vi "Scope_5782.vi"() -> ()   [LabVIEW 2013]
uses:
  <vilib>/userdefined/High Color/nirio_resource_hc.ctl
  FPGA/DataMode.ctl
  <vilib>/Analysis/4window.llb/windowTd.ctl
  Host/Scope/controls/power_spectrum_unit.ctl
  Host/Scope5782/Scope/controls/5782_trigger_type.ctl
  Host/Scope/controls/Data_calc_mode.ctl
  Host/Scope/controls/Data_display_mode.ctl
  Host/Scope/controls/Graph_references.ctl
  Host/Scope/controls/graph_controls.ctl
  Host/Scope/controls/Channel_select.ctl
  Host/Scope5782/Config/FPGAref_5782.ctl
  Host/Communication/response.ctl
  Host/Communication/driver_status.ctl
  Host/Communication/Driver/RemoteConnection/RemoteReferences.ctl
  Host/Communication/Driver/TcpServerDriver/TcpServerDriver.lvclass
  Host/Scope/controls/ScopeMode.ctl
  FPGA/fpga_settings.ctl
  Host/Communication/global_stop.vi
  <vilib>/FPGAPlugInAG/PXIe-7975R/niLvFpga_Open_PXIe-7975R.vi
  <vilib>/rvi/interface/common/dynamic/niFpgaDynamicAddResources.vi
  <vilib>/rvi/interface/common/niFpgaWaitOnOcc.vi
  <vilib>/Utility/error.llb/Error Cluster From Error Code.vi
  <vilib>/rvi/errors/niLvFpgaAdjustHostInterfaceError.vi
  <vilib>/FPGAPlugInAG/Dynamic/niLvFpga_Close_Dynamic.vi
  <vilib>/rvi/interface/nirviOpenFPGA/nirviOpenFPGA.xnode
  FPGA Bitfiles/mixer_FPGATarget2_FPGAmain5782_W462Q9ePIkg.lvbitx
  <vilib>/rvi/interface/nirviReadWriteControl/nirviReadWriteControl.xnode
  <vilib>/rvi/FXPMathLib/FxpInterpret/XNode/nifxpmath_Interpret.xnode
  <vilib>/rvi/interface/nirviCloseFPGA/nirviCloseFPGA.xnode
  Host/Utilities/Ticker/Ticker.lvclass
  NiFpgaLv.dll
  <vilib>/rvi/interface/Simulation/niFpgaSimulationCallBeginRW.vi
  Host/Communication/Driver/RemoteConnection/RemoteConnection.lvclass
  <vilib>/Analysis/NI_AALPro.lvlib
panel:
  in  "deltaF":bool
  in  "b":fxp<+/-,16,2>
  in  "a":fxp<+/-,16,2>
  in  "Fequency [kHz]":dbl format="%#_8g"
  in  "#bins":i32=1 min=1 max=16
  in  "ch1 DC offset":dbl caption="DC offset\nChannel 1"
  in  "ch0 DC offset":dbl caption="DC offset\nChannel 0"
  in  "Output delay delta":dbl(slide) scale=0.0..6.0
  in  "Output delay":dbl(slide) scale=0.0..6.0
  in  "Chart length":i32=200000
  in  "Trigmode":enum32{"Triggered", "Continuous"}(radio)
  in  "Refence for phase":T1
  in  "Graph_refs":T2
  out "Lower chart":dbl[][](graph)
  out "Upper chart":dbl[][](graph)
  out "Lower graph":i16[][](graph)
  in  "Buffer":T4
  in  "Display":T5
  in  "Output mixer fequency [MHz]":dbl
  in  "Trigger":T6
  in  "Ch1 Q":bool
  in  "Ch1 I":bool
  in  "Ch0 Q":bool
  in  "Ch0 I":bool
  in  "Ch1":bool
  in  "Ch0":bool
  out "stop 2":bool
  in  "Zoom freq X":bool
  in  "Zoom freq Y":bool
  in  "Zoom time Y":bool
  in  "Zoom time X":bool
  in  "Unit":T7
  in  "Window":T8=1 items=["Rectangle"=0, "Hanning"=1, "Hamming"=2, "Blackman-Harris"=3, "Exact Blackman"=4, "Blackman"=5, "Flat Top"=6, "4 Term B-Harris "=7, "7 Term B-Harris"=8, "Low Sidelobe"=9, "Blackman Nuttall"=11, "Triangle"=30, "Bartlett-Hanning"=31, "Bohman"=32, "Parzen"=33, "Welch"=34, "Kaiser"=60, "Dolph-Chebyshev"=61, "Gaussian"=62]
  in  "Samples per 5782 record":i32
  in  "Phase offset (deg)":dbl
  in  "Fequency [MHz]":dbl format="%#_8g"
  in  "Mode":T9
  in  "Mixer freq [MHz]":dbl
  out "freqdata":cluster{"f0":dbl, "df":dbl, "magnitude":dbl[]}[](graph)
  in  "Rumode":bool
  in  "Singleshot":bool
  out "error IO":errorcluster
  in  "stop":bool
  in  "resource name":T10="RIO0"
  out "Clocking Option Configured?":bool
  out "Configured?":bool
  # "FPGA setup"
  # "V"
  # "V"
  # "Output delay"
  # "ns"
  # "Auto Zoom"
  # "Output delay delta"
  # "ps"
  # "5782"
  # "Amplitude modulation"
  # "Simulated data"
  # "FFT"
  # "Auto Zoom"
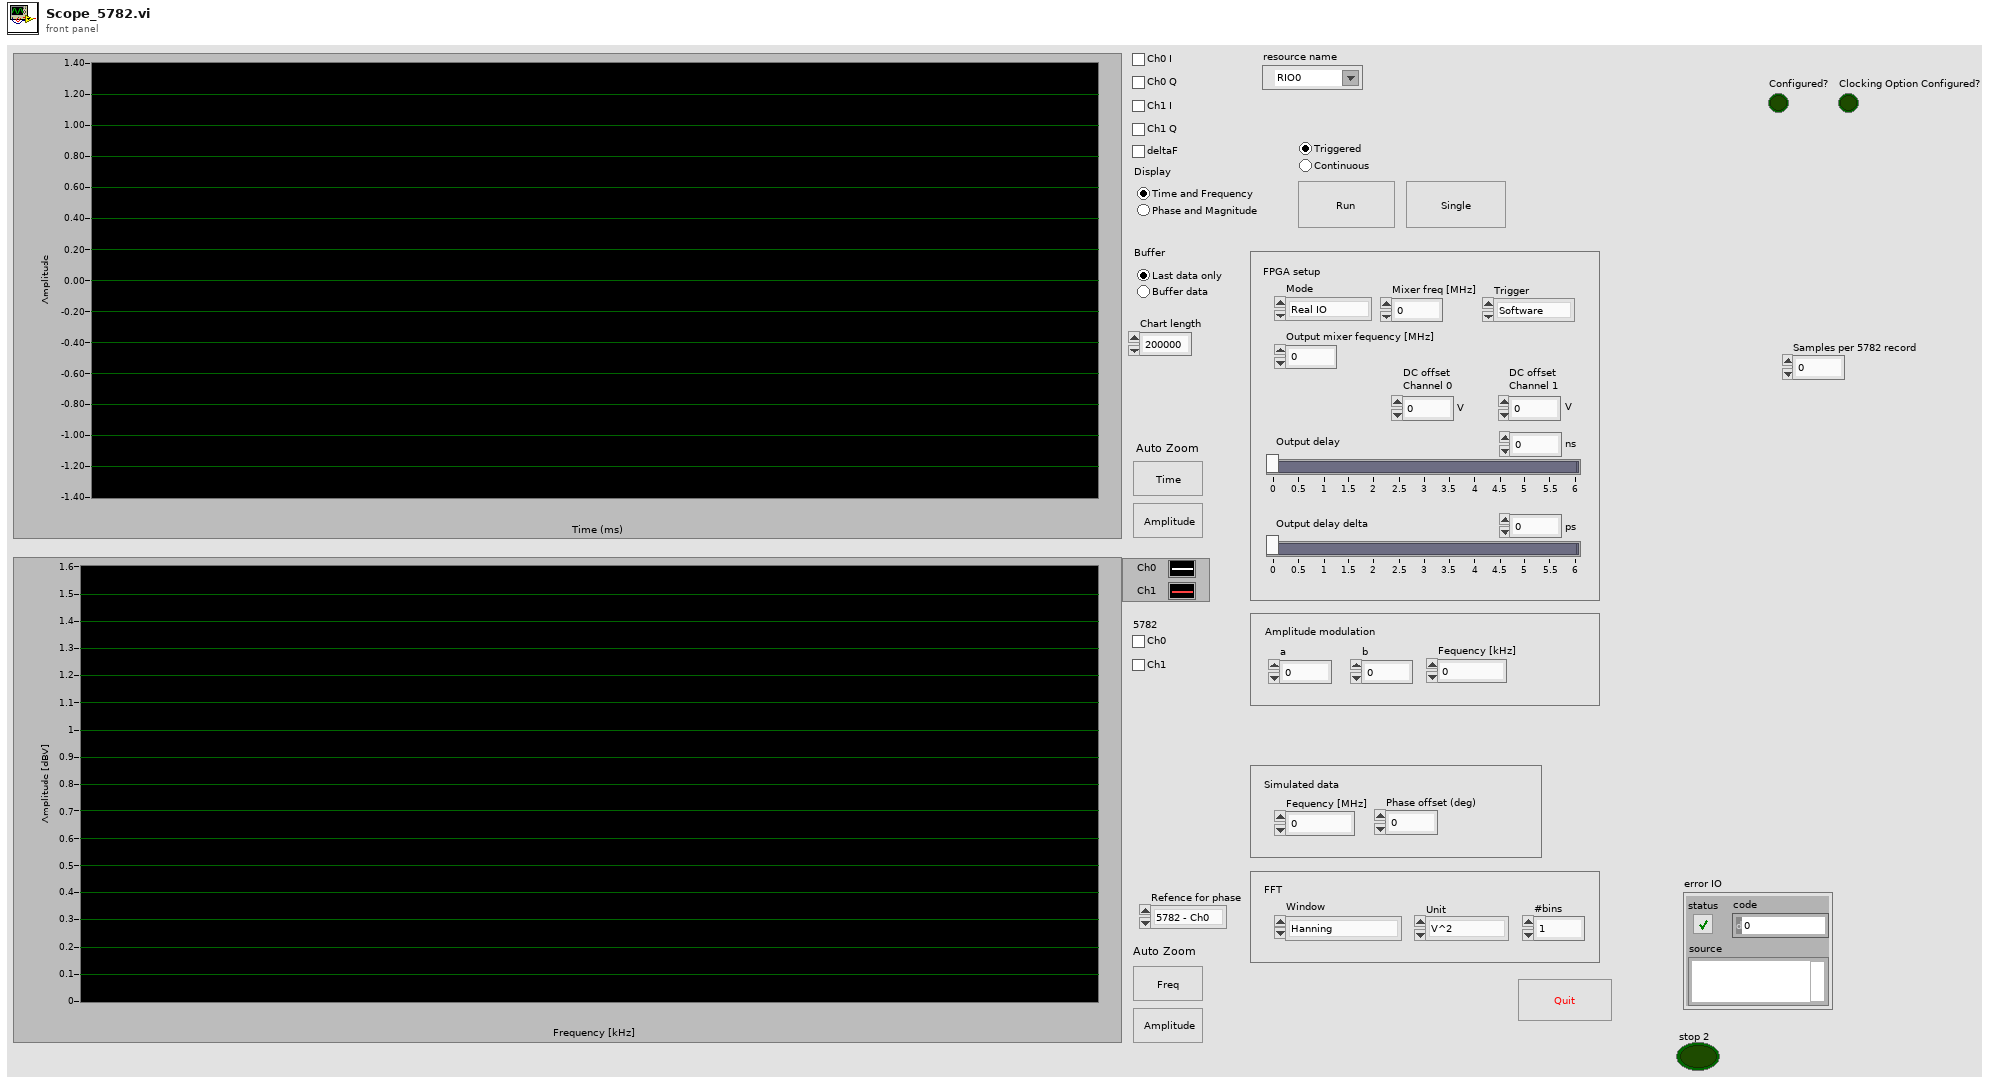
[diagram p1: front panel]
types:
  T1 = typedef "Channel_select.ctl" = enum16{"5782 - Ch0", "5782 - Ch1"}
  T2 = typedef "Graph_references.ctl" = cluster{"upper":T3, "lower":T3, "Freq graph":refnum<vi>}
  T3 = typedef "graph_controls.ctl" = cluster{"Graph":refnum<vi>, "Time btn":refnum<vi>, "Amplitude btn":refnum<vi>, "Chart":refnum<vi>}
  T4 = typedef "Data_display_mode.ctl" = enum32{"Last data only", "Buffer data"}
  T5 = typedef "Data_calc_mode.ctl" = enum32{"Time and Frequency", "Phase and Magnitude"}
  T6 = typedef "5782_trigger_type.ctl" = enum16{"Software", "Trigger input"}
  T7 = typedef "power_spectrum_unit.ctl" = enum16{"V^2", "V", "dBV"}
  T8 = typedef "NI_AALPro.lvlib/windowTd.ctl" = u32
  T9 = typedef "DataMode.ctl" = enum16{"Real IO", "Simulated"}
  T10 = typedef "nirio_resource_hc.ctl" = tag
  T11 = typedef "RemoteConnection.lvclass/RemoteReferences.ctl" = cluster{"a":refnum<vi>, "b":refnum<vi>, "fm":refnum<vi>}
  T12 = typedef "response.ctl" = cluster{"driver status":T13, "Sender":string, "Type":i32, "Variant":variant}
  T13 = typedef "driver_status.ctl" = enum16{"Normal", "Startup", "Connection lost", "Reconnected", "Timeout", "Idle", "Busy"}
  T14 = typedef "FPGAref_5782.ctl" = refnum<k20>
  T15 = enum8{"Internal Clock PLL Off", "Internal Clock PLL On (REF IN)", "External Clock (CLK_IN)", "Internal Clock PLL On (IoModSyncClk)"}
  T16 = typedef "message_queue.ctl" = refnum<queue>
  T17 = typedef "scope_params_5782.ctl" = cluster{"scope mode":T18, "ticker":refnum<class "Ticker.lvclass">, "samples per record":i32, "FPGA ref":T14, "data mode":T9, "5782 Trigger":T6, "Chart length":i32, "RemoteConnection":refnum<class "RemoteConnection.lvclass">, "last phase":dbl[]}
  T18 = typedef "ScopeMode.ctl" = enum16{"Stopped", "Single", "Running", "Continuous"}
  T19 = typedef "fpga_settings.ctl" = enum16{"Feedback Enable", "New FIR coeffs", "FIR shift", "Enable filter", "Set Downsample", "Downsample", "CIC Gain", "Record length", "Trigger samples", "Quiet time", "a_am", "b_am", "Use fixed delay", "fixed sin_fi", "fixed cos_fi", "Ki*Tau", "Kp", "Kd_Tau", "Fi_start", "Fi_delta", "DC_offs 0", "DC_offs 1"}
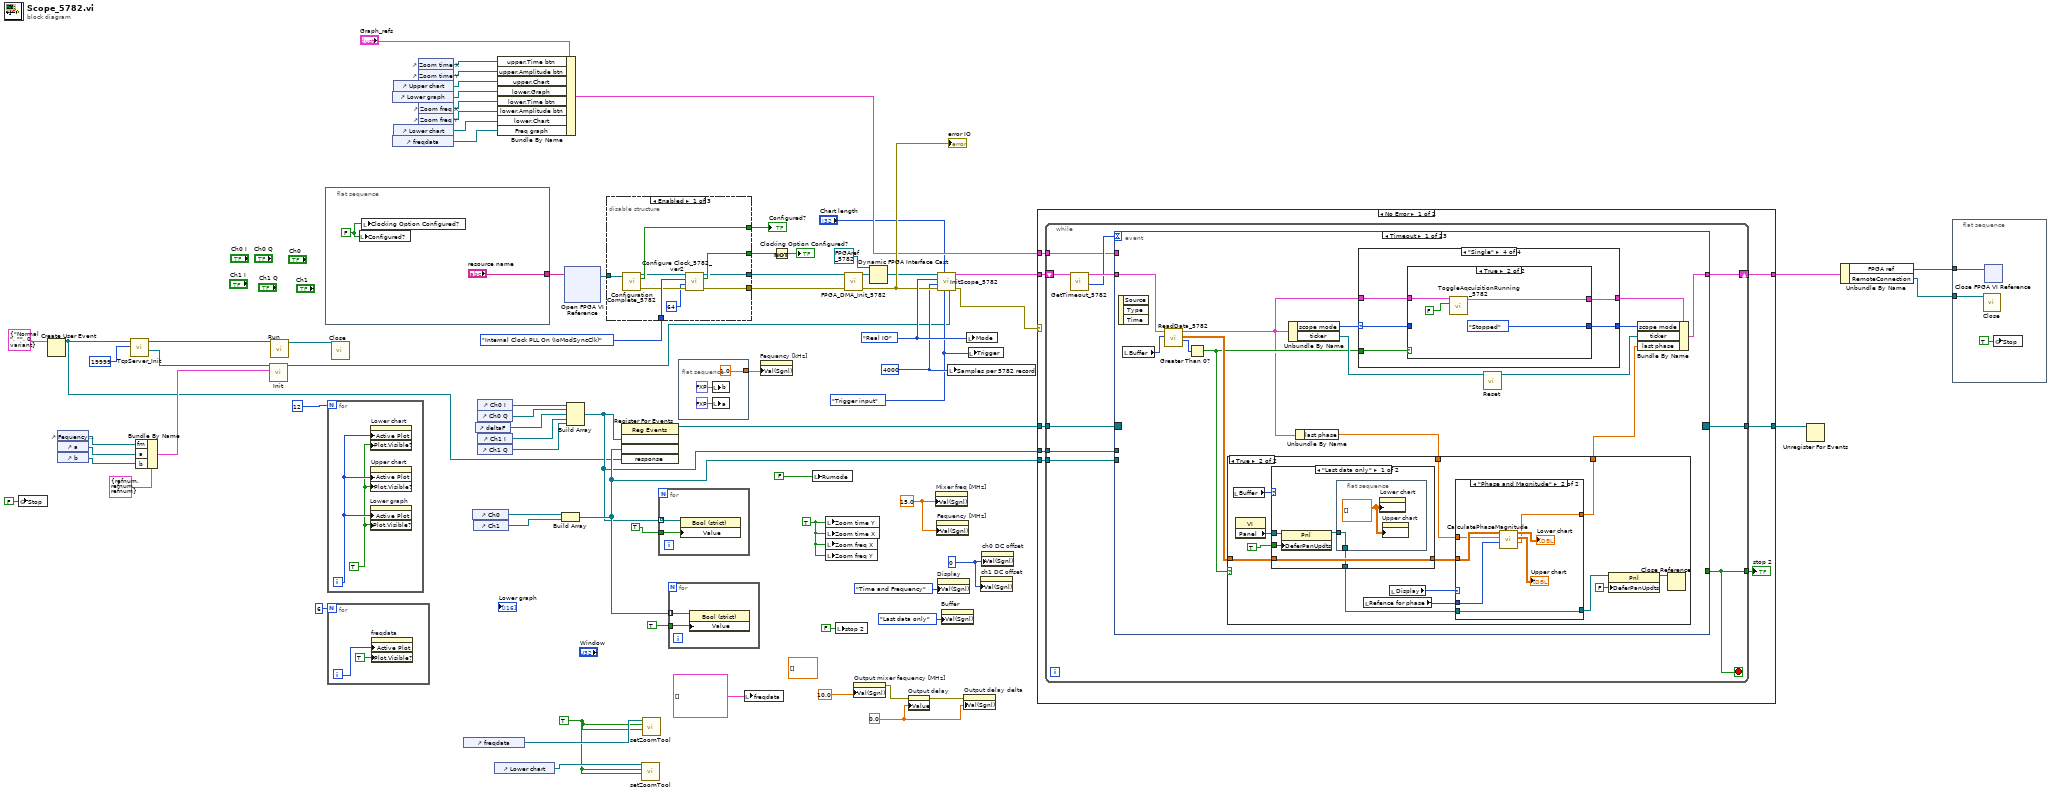
[diagram p0: block diagram]
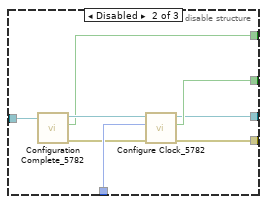
[diagram p2: hidden frame]
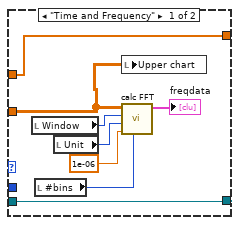
[diagram p6: hidden frame]
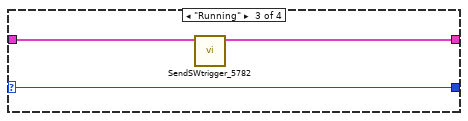
[diagram p9: hidden frame]
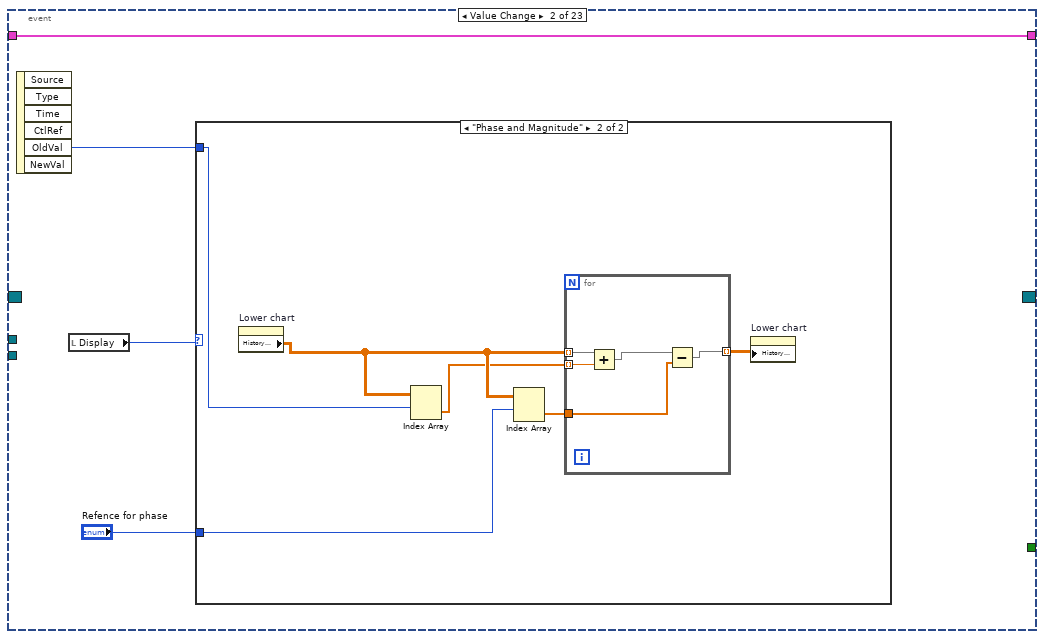
[diagram p11: hidden frame]
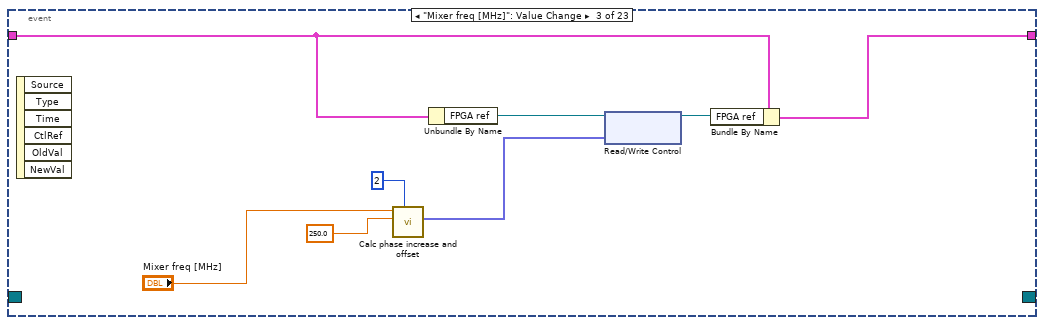
[diagram p13: hidden frame]
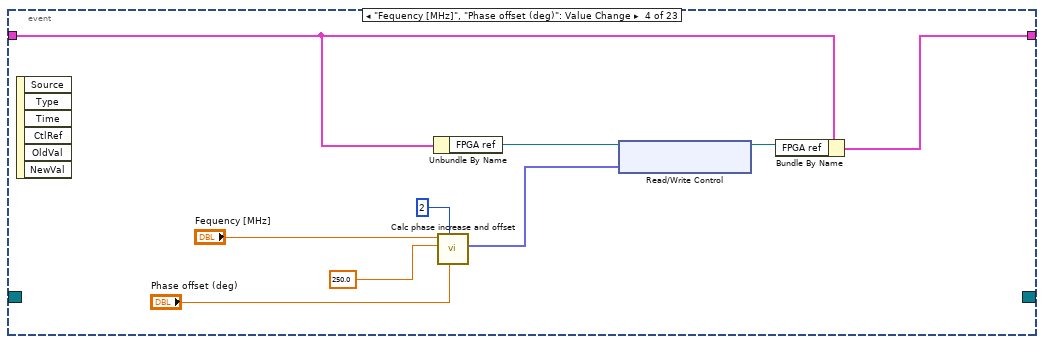
[diagram p14: hidden frame]
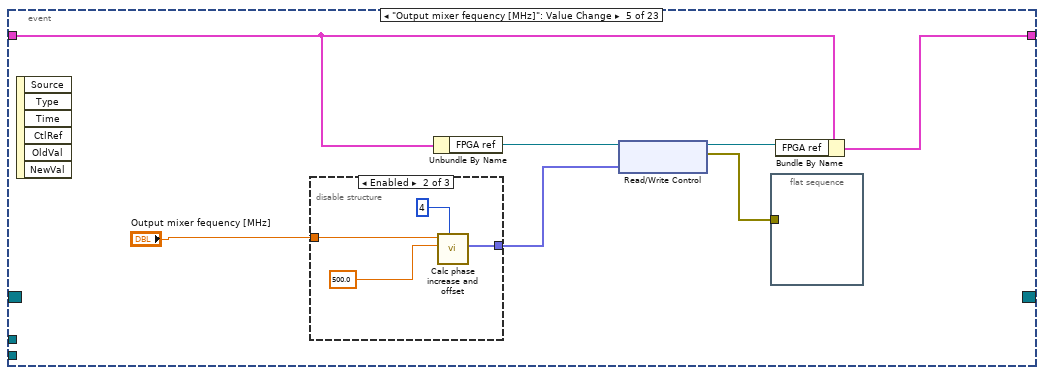
[diagram p15: hidden frame]
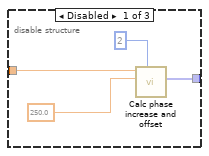
[diagram p16: hidden frame]
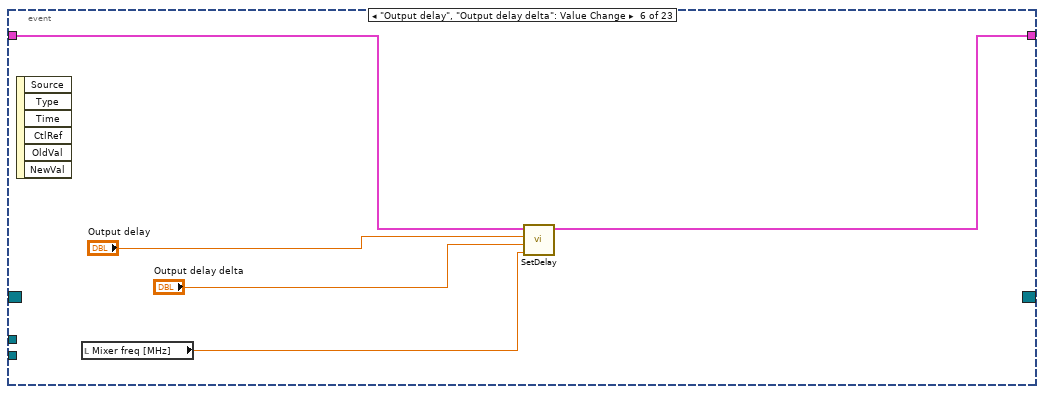
[diagram p18: hidden frame]
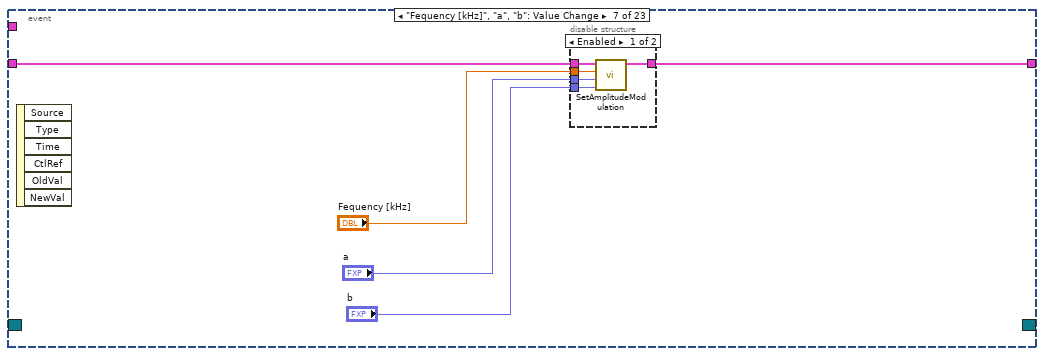
[diagram p19: hidden frame]
diagram:
  w26 = i16 0 ("Value (Signaling)")
  w27 = 0.0 ("Value (Signaling)")
  w49 = 5782_trigger_type."Trigger input" ("Trigger")
  w2 = TRUE ("Zoom  X")
  w62 = TRUE ("Rumode")
  w61 = DataMode."Real IO" ("Mode")
  w50 = 4000 ("Samples to aqcuire")
  (unwired) dbl[][] [] ("Timedata")
  w72 = 15.0 ("Mixer requency [MHz]")
  n1 = global write "global_stop.vi" "Stop"(FALSE ("Stop")) -> ()
  n2 = Create User Event(user event datatype=T12 {"driver status"=enum."Normal", "Sender"="", "Type"=0, "Variant"=variant} ("response")) -> (user event=w9:refnum<user-event>)  [unwired: 1 in, 1 out]
  n3 = control-ref of="Fequency [kHz]"() -> (w12:refnum<vi>)
  n4 = control-ref of="a"() -> (w11:refnum<vi>)
  n5 = control-ref of="b"() -> (w10:refnum<vi>)
  n6 = call "TcpServer_Init.vi"("local port"=u16 19999, "response event"=w9) -> ("Message queue"=w19:T16, "TcpServerDriver"=w16:refnum<class "TcpServerDriver.lvclass">)  [unwired: 8 in]
  n7 = Bundle By Name(cluster=T11 {"a"=refnum, "b"=refnum, "fm"=refnum} ("refs"), "fm"=w12, "a"=w11, "b"=w10) -> (w13:T11)
  n8 = call "Init.vi"("refs"=w13, "server queue"=w19) -> ("RemoteConnection"=w8:refnum<class "RemoteConnection.lvclass">)  [unwired: 9 in]
  n9 = call-dynamic "Run.vi"("BaseDriver in"=w16) -> ("BaseDriver out"=w17:refnum<class "TcpServerDriver.lvclass">)  [unwired: 9 in, 1 out]
  n10 = flat-sequence {
    tunnel: ["resource name"] -> w63
    frame #0 {
      w76 = FALSE ("Trigger Acquisition")
      n11 = local write "Configured?"(w76) -> ()
      n12 = local write "Clocking Option Configured?"(w76) -> ()
    }
  }
  n13 = for {
    N: 12 -> [_]
    i -> [w79]
    w78 = TRUE ("Plot.Visible")
    n14 = property on="Lower graph" class="WFGraph (strict)"("Active Plot"=w79, "Plot.Visible?"=w78) -> ()  [unwired: 2 in, 2 out]
    n15 = property on="Lower chart" class="WFChart (strict)"("Active Plot"=w79, "Plot.Visible?"=w78) -> ()  [unwired: 2 in, 2 out]
    n16 = property on="Upper chart" class="WFChart (strict)"("Active Plot"=w79, "Plot.Visible?"=w78) -> ()  [unwired: 2 in, 2 out]
  }
  n17 = for {
    N: 6 -> [_]
    i -> [w80]
    n18 = property on="freqdata" class="WFGraph (strict)"("Active Plot"=w80, "Plot.Visible?"=TRUE ("Plot.Visible")) -> ()  [unwired: 2 in, 2 out]
  }
  n19 = call-dynamic "Close.vi"("BaseDriver in"=w17) -> ()  [unwired: 9 in, 2 out]
  n20 = control-ref of="Lower graph"() -> (w43:refnum<vi>)
  n21 = control-ref of="freqdata"() -> (w39:refnum<vi>)
  n22 = control-ref of="Upper chart"() -> (w44:refnum<vi>)
  n23 = control-ref of="Lower chart"() -> (w40:refnum<vi>)
  n24 = control-ref of="Zoom time X"() -> (w46:refnum<vi>)
  n25 = control-ref of="Zoom time Y"() -> (w45:refnum<vi>)
  n26 = control-ref of="Zoom freq X"() -> (w42:refnum<vi>)
  n27 = control-ref of="Zoom freq Y"() -> (w41:refnum<vi>)
  n28 = control-ref of="freqdata"() -> (w52:refnum<vi>)
  n29 = control-ref of="Ch0"() -> (w58:refnum<vi>)
  n30 = control-ref of="Ch1"() -> (w59:refnum<vi>)
  n31 = control-ref of="deltaF"() -> (w1:refnum<vi>)
  n32 = control-ref of="Ch0 I"() -> (w54:refnum<vi>)
  n33 = control-ref of="Ch0 Q"() -> (w55:refnum<vi>)
  n34 = control-ref of="Ch1 I"() -> (w56:refnum<vi>)
  n35 = control-ref of="Ch1 Q"() -> (w57:refnum<vi>)
  n36 = control-ref of="Lower chart"() -> (w3:refnum<vi>)
  n37 = Bundle By Name(cluster="Graph_refs", "upper.Time btn"=w46, "upper.Amplitude btn"=w45, "upper.Chart"=w44, "lower.Graph"=w43, "lower.Time btn"=w42, "lower.Amplitude btn"=w41, "lower.Chart"=w40, "Freq graph"=w39) -> (w38:T2)
  n38 = Build Array(w58, w59) -> (w65:refnum<vi>[])
  n39 = xnode "Open FPGA VI Reference"("resource name"=w63) -> ("FPGA VI Reference Out"=w32:refnum<k20>)  [unwired: 1 in, 1 out]
  n40 = Build Array(w54, w55, w1, w56, w57) -> (w53:refnum<vi>[])
  n41 = disable-structure shown="Enabled" {
    disable-tunnel: [w90 w98 _] -> w34
    disable-tunnel: T15."Internal Clock PLL On (IoModSyncClk)" ("Clock Source") -> [w89 w97 _]
    disable-tunnel: [w87 w95 _] -> w33
    disable-tunnel: [w86 w92 w99] -> w25
    disable-tunnel: w32 -> [w83 w94 w99]
    disable-tunnel: [w85 w91 _] -> w30
    frame Enabled {
      n42 = call "Configuration Complete_5782.vi"("FPGA VI Reference in"=w83) -> ("error out"=w88:errorcluster, "Configured?"=w85:bool, "FPGA VI Reference out"=w84:refnum<k20>)  [unwired: 8 in]
      n43 = call "Configure Clock_5782_ver2.vi"("error in"=w88, "User Data 1"=u8 64, "Clock Source"=w89, "FPGA VI Reference"=w84) -> ("error out"=w87:errorcluster, "Configuration Error"=w90:bool, "FPGA VI Reference out"=w86:refnum<k20>)  [unwired: 5 in]
    }
    frame Disabled {
      n44 = call "Configuration Complete_5782.vi"("FPGA VI Reference in"=w94) -> ("error out"=w96:errorcluster, "Configured?"=w91:bool, "FPGA VI Reference out"=w93:refnum<k20>)  [unwired: 8 in]
      n45 = call "Configure Clock_5782.vi"("error in"=w96, "Clock Source"=w97, "FPGA VI Reference in"=w93) -> ("error out"=w95:errorcluster, "Configuration Error"=w98:bool, "FPGA VI Reference Out"=w92:T14)  [unwired: 6 in]
    }
    frame Disabled {
    }
  }
  "Configured?" <- w30
  n46 = register-events(w53, w65, w9) -> (reference out=w69:refnum<event-registration>)  [unwired: 2 in, 1 out]
  n47 = call "setZoomTool.vi"("Zoom Y"=w2, "Zoom  X"=w2, "reference"=w3) -> ()  [unwired: 9 in]
  n48 = call "setZoomTool.vi"("Zoom Y"=w2, "Zoom  X"=w2, "reference"=w52) -> ()  [unwired: 9 in]
  n49 = for {
    tunnel: w53 -> [w101] mode=indexing
    tunnel: TRUE ("Rumode") -> [w100]
    n50 = property class="Bool (strict)"(reference=w101, "Value"=w100) -> ()  [unwired: 1 in, 2 out]
  }
  n51 = for {
    tunnel: w65 -> [w103] mode=indexing
    tunnel: TRUE ("Rumode") -> [w102]
    n52 = property class="Bool (strict)"(reference=w103, "Value"=w102) -> ()  [unwired: 1 in, 2 out]
  }
  n53 = flat-sequence {
    tunnel: [1.0 ("Value (Signaling)")] -> w24
    frame #0 {
      n54 = local write "b"(fxp<+/-,16,2> 0.0 ("b")) -> ()
      n55 = local write "a"(fxp<+/-,16,2> 1.0 ("a")) -> ()
    }
  }
  n56 = local write "freqdata"(cluster{"f0":dbl, "df":dbl, "magnitude":dbl[]}[] [] ("freqdata")) -> ()
  n57 = property on="Fequency [kHz]" class="DigNum (strict)"("Val(Sgnl)"=w24) -> ()  [unwired: 2 in, 2 out]
  n58 = Not(x=w34) -> (.not. x?=→"Clocking Option Configured?":bool)
  n59 = local write "Rumode"(FALSE ("Rumode")) -> ()
  n60 = local write "Zoom time Y"(w62) -> ()
  n61 = local write "Zoom time X"(w62) -> ()
  n62 = local write "Zoom freq X"(w62) -> ()
  n63 = local write "Zoom freq Y"(w62) -> ()
  n64 = local write "stop 2"(FALSE ("stop 2")) -> ()
  n65 = call "FPGA_DMA_Init_5782.vi"("error in (no error)"=w33, "FPGA VI Reference"=w25) -> ("error out"=w51:errorcluster, "FPGA VI Out"=w22:refnum<k20>)  [unwired: 7 in, 1 out]
  "error IO" <- w51
  n66 = property on="Output mixer fequency [MHz]" class="DigNum (strict)"("Val(Sgnl)"=10.0 ("Mixer requency [MHz]")) -> (error out=w28:errorcluster)  [unwired: 2 in, 1 out]
  n67 = Dynamic FPGA Interface Cast(Session In=T14 refnum ("FPGA ref"), Type=w22) -> (Session Out=w21:T14)
  n68 = property on="Output delay" class="Slide (strict)"(error in=w28, "Value"=w27) -> (error out=w29:errorcluster)  [unwired: 1 in, 1 out]
  n69 = property on="Mixer freq [MHz]" class="DigNum (strict)"("Val(Sgnl)"=w72) -> ()  [unwired: 2 in, 2 out]
  n70 = property on="Fequency [MHz]" class="DigNum (strict)"("Val(Sgnl)"=w72) -> ()  [unwired: 2 in, 2 out]
  n71 = call "InitScope_5782.vi"("RemoteConnection"=w8, "Trigger"=w49, "Chart length"="Chart length", "error in"=w51, "Samples Per Trigger"=w50, "data mode"=w61, "FPGA ref"=w21) -> ("error out"=w7:errorcluster, "scope params"=w75:T17)  [unwired: 3 in]
  n72 = property on="Display" class="RadioBtnsControl (strict)"("Val(Sgnl)"=Data_calc_mode."Time and Frequency" ("Value (Signaling)")) -> ()  [unwired: 2 in, 2 out]
  n73 = property on="Buffer" class="RadioBtnsControl (strict)"("Val(Sgnl)"=enum32{"Last data only", "Buffer data"}."Last data only" ("Value (Signaling)")) -> ()  [unwired: 2 in, 2 out]
  n74 = local write "Samples per 5782 record"(w50) -> ()
  n75 = property on="Output delay delta" class="Slide (strict)"(error in=w29, "Val(Sgnl)"=w27) -> ()  [unwired: 1 in, 2 out]
  n76 = local write "Mode"(w61) -> ()
  n77 = local write "Trigger"(w49) -> ()
  n78 = property on="ch1 DC offset" class="DigNum (strict)"("Val(Sgnl)"=w26) -> ()  [unwired: 2 in, 2 out]
  n79 = property on="ch0 DC offset" class="DigNum (strict)"("Val(Sgnl)"=w26) -> ()  [unwired: 2 in, 2 out]
  n80 = case shown="No Error" w7 {
    tunnel: w75 -> [w114 w396]
    tunnel: [w113 w396] -> w4
    tunnel: w69 -> [w112 w395]
    tunnel: [w111 w395] -> w68
    tunnel: w53 -> [w110 _]
    tunnel: w65 -> [w109 _]
    tunnel: w38 -> [w107 _]
    frame No Error {
      n81 = while {
        shift-right: [w124] -> w113
        shift-left: w114 -> [w123]
        tunnel: w112 -> [w120]
        tunnel: [w119] -> w111
        tunnel: w110 -> [w118]
        tunnel: w109 -> [w117]
        tunnel: [w116] -> w108
        tunnel: w107 -> [w115]
        stop <- w116 stop-if-true
        n82 = call "GetTimeout_5782.vi"("scope in"=w123) -> ("Time left"=w121:i32, "scope out"=w122:T17)  [unwired: 9 in]
        n83 = event shown="[0] Timeout" {
          selector: w120 -> [_ _ _ _ _ _ _ _ _ _ _ _ _ _ _ _ _ _ _ _ _ _ _]
          dyn-events: [_ _ _ _ _ _ _ _ _ _ _ _ _ _ _ _ _ _ _ _ _ _ _] -> w119
          timeout: w121 -> [_ _ _ _ _ _ _ _ _ _ _ _ _ _ _ _ _ _ _ _ _ _ _]
          tunnel: [_ _ _ _ _ _ _ _ _ _ _ _ _ _ _ _ _ "stop" _ _ _ _ _] -> w116
          tunnel: w122 -> [w133 w198 w216 w222 w231 w246 w251 w271 w285 w289 w293 w296 w308 w317 w342 w347 w349 w355 w362 w372 w376 w382 w385]
          tunnel: [w136 w198 w214 w221 w230 w245 w250 w270 w284 w288 w292 w295 w300 w314 w342 w347 w348 w355 w362 w372 w376 w382 w383] -> w124
          tunnel: w118 -> [_ _ _ _ _ _ _ _ _ _ _ _ _ _ w341 _ _ _ _ _ _ _ _]
          tunnel: w117 -> [_ _ _ _ _ _ _ _ _ _ _ _ _ _ _ w345 _ _ _ _ _ _ _]
          tunnel: w115 -> [_ _ _ _ _ _ _ _ _ _ _ _ _ _ _ _ _ _ _ _ _ _ w392]
          event Timeout {
            n84 = event-data() -> ()  [unwired: 1 in, 3 out]
            n85 = local read "Buffer"() -> (w128:T4)
            n86 = call "ReadData_5782.vi"("Buffer mode"=w128, "scope params"=w133) -> ("Num elements"=w130:i32, "data"=w131:dbl[][], "scope params out"=w127:T17)  [unwired: 7 in]
            n87 = Greater Than 0?(x=w130) -> (x > 0?=w129:bool)
            n88 = Unbundle By Name(w127) -> ("scope mode"=w135:T18, "ticker"=w138:refnum<class "Ticker.lvclass">)
            n89 = Unbundle By Name(w127) -> ("last phase"=w126:dbl[])
            n90 = case shown="True" w129 {
              tunnel: w131 -> [_ w149]
              tunnel: w126 -> [w139 w141]
              tunnel: [w139 w140] -> w125
              frame False {
              }
              frame True {
                n91 = local read "Buffer"() -> (w151:T4)
                n92 = property class="VI"() -> ("Panel"=w144:refnum<vi>)  [unwired: 2 in, 2 out]
                n93 = case shown="\"Last data only\"" w151 {
                  tunnel: w149 -> [w157 w161]
                  tunnel: [w157 w161] -> w150
                  tunnel: w144 -> [w156 w160]
                  tunnel: TRUE ("Defer Panel Updates") -> [w154 _]
                  tunnel: [w153 w160] -> w142
                  frame "Last data only" {
                    n94 = property class="Pnl"(reference=w156, "DeferPanUpdts"=w154) -> (reference out=w155:refnum<vi>)  [unwired: 1 in, 1 out]
                    n95 = flat-sequence {
                      tunnel: w155 -> [w158]
                      tunnel: [w158] -> w153
                      frame #0 {
                        w159 = dbl[][] [] ("History Data")
                        n96 = property on="Lower chart" class="WFChart (strict)"("History Data"=w159) -> ()  [unwired: 2 in, 2 out]
                        n97 = property on="Upper chart" class="WFChart (strict)"("History Data"=w159) -> ()  [unwired: 2 in, 2 out]
                      }
                    }
                  }
                  frame "Buffer data" {
                  }
                }
                n98 = local read "Refence for phase"() -> (w148:T1)
                n99 = local read "Display"() -> (w152:T5)
                n100 = case shown="\"Phase and Magnitude\"" w152 {
                  tunnel: w150 -> [w165 w176]
                  tunnel: w148 -> [_ w173]
                  tunnel: [w164 w172] -> w146
                  tunnel: w142 -> [w164 w172]
                  tunnel: w141 -> [w162 w171]
                  tunnel: [w162 w170] -> w140
                  frame "Time and Frequency" {
                    n101 = local read "Window"() -> (w166:T8)
                    n102 = local read "#bins"() -> (w163:i32)
                    n103 = local read "Unit"() -> (w167:T7)
                    n104 = local write "Upper chart"(w165) -> ()
                    n105 = call "calc FFT.vi"("#bins"=w163, "dt"=1e-06, "Unit"=w167, "Window"=w166, "data"=w165) -> ("Power Spectrum / PSD"=→"freqdata":cluster{"f0":dbl, "df":dbl, "magnitude":dbl[]}[])  [unwired: 6 in]
                  }
                  frame "Phase and Magnitude" {
                    n106 = call "CalculatePhaseMagnitude.vi"("phase reference channel"=w173, "previous phase"=w171, "data"=w176) -> ("last phase"=w170:dbl[], "Magnitude"=→"Upper chart":dbl[][], "Phase"=→"Lower chart":dbl[][])  [unwired: 6 in]
                  }
                }
                n107 = property class="Pnl"(reference=w146, "DeferPanUpdts"=FALSE ("Defer Panel Updates")) -> (reference out=w145:refnum<vi>)  [unwired: 1 in, 1 out]
                n108 = Close Reference(reference=w145) -> ()  [unwired: 1 in, 1 out]
              }
            }
            n109 = case shown="\"Single\"" w135 {
              selector: w135 -> [w178 w180 w183 w184]
              tunnel: [w178 w180 w183 w188] -> w134
              tunnel: w127 -> [w177 w179 w182 w186]
              tunnel: [w177 w179 w181 w185] -> w132
              tunnel: w129 -> [_ _ _ w187]
              frame "Stopped" {
              }
              frame "Continuous" {
              }
              frame "Running" {
                n110 = call "SendSWtrigger_5782.vi"("scope in"=w182) -> ("scope out"=w181:T17)  [unwired: 9 in, 1 out]
              }
              frame "Single" {
                n111 = case shown="True" w187 {
                  tunnel: [w189 ScopeMode."Stopped" ("scope mode")] -> w188
                  tunnel: w186 -> [w190 w193]
                  tunnel: [w190 w192] -> w185
                  tunnel: w184 -> [w189 _]
                  frame False {
                  }
                  frame True {
                    n112 = call "ToggleAqcuisitionRunning_5782.vi"("Acquisition running"=FALSE, "scope in"=w193) -> ("scope out"=w192:T17)  [unwired: 8 in, 1 out]
                  }
                }
              }
            }
            n113 = call "Reset.vi"("Ticker in"=w138) -> ("Ticker out"=w137:refnum<class "Ticker.lvclass">)  [unwired: 9 in, 1 out]
            n114 = Bundle By Name(cluster=w132, "scope mode"=w134, "ticker"=w137, "last phase"=w125) -> (w136:T17)
          }
          event Value Change {
            n115 = event-data() -> ("OldVal"=w195:T1)  [unwired: 1 in, 5 out]
            n116 = local read "Display"() -> (w196:T5)
            n117 = case shown="\"Phase and Magnitude\"" w196 {
              tunnel: "Refence for phase" -> [_ w203]
              tunnel: w195 -> [_ w201]
              frame "Time and Frequency", Default {
              }
              frame "Phase and Magnitude" {
                n118 = property on="Lower chart" class="WFChart (strict)"() -> ("History Data"=w202:dbl[][])  [unwired: 2 in, 2 out]
                n119 = Index Array(array=w202, index (row)=w201) -> (element=w200:dbl[])  [unwired: 1 in]
                n120 = Index Array(array=w202, index (row)=w203) -> (element=w204:dbl[])  [unwired: 1 in]
                n121 = for {
                  tunnel: w202 -> [w207] mode=indexing
                  tunnel: w204 -> [w209]
                  tunnel: [w208] -> w199 mode=indexing
                  tunnel: w200 -> [w206] mode=indexing
                  n122 = Add(x=w207, y=w206) -> (x+y=w205:dbl[])
                  n123 = Subtract(x=w205, y=w209) -> (x-y=w208:dbl[])
                }
                n124 = property on="Lower chart" class="WFChart (strict)"("History Data"=w199) -> ()  [unwired: 2 in, 2 out]
              }
            }
          }
          event "Mixer freq [MHz]": Value Change {
            n125 = event-data() -> ()  [unwired: 1 in, 6 out]
            n126 = call "Calc phase increase and offset.vi"("# of DDS"=2, "fclk (MHz)"=250.0 ("fclk (800MHz)"), "f_generated (MHz)"="Mixer freq [MHz]") -> ("Phase out"=w210:fxp<+,64,64>[])  [unwired: 6 in, 2 out]
            n127 = Unbundle By Name(w216) -> ("FPGA ref"=w217:T14)
            n128 = xnode "Read/Write Control"("FPGA VI Reference In"=w217, "Phase 5782"=w210) -> ("FPGA VI Reference Out"=w215:T14)  [unwired: 1 in, 1 out]
            n129 = Bundle By Name(cluster=w216, "FPGA ref"=w215) -> (w214:T17)
          }
          event "Fequency [MHz]", "Phase offset (deg)": Value Change {
            n130 = event-data() -> ()  [unwired: 1 in, 6 out]
            n131 = Unbundle By Name(w222) -> ("FPGA ref"=w224:T14)
            n132 = call "Calc phase increase and offset.vi"("Phase offset (deg)"="Phase offset (deg)", "# of DDS"=2, "fclk (MHz)"=250.0 ("fclk (800MHz)"), "f_generated (MHz)"="Fequency [MHz]") -> ("Phase out"=w218:fxp<+,64,64>[])  [unwired: 5 in, 2 out]
            n133 = xnode "Read/Write Control"("FPGA VI Reference In"=w224, "Simulated phase 5782"=w218) -> ("FPGA VI Reference Out"=w223:T14)  [unwired: 1 in, 1 out]
            n134 = Bundle By Name(cluster=w222, "FPGA ref"=w223) -> (w221:T17)
          }
          event "Output mixer fequency [MHz]": Value Change {
            n135 = event-data() -> ()  [unwired: 1 in, 6 out]
            n136 = disable-structure shown="Enabled" {
              disable-tunnel: [w235 w239 _] -> w227
              disable-tunnel: "Output mixer fequency [MHz]" -> [w234 w238 _]
              frame Disabled {
                n137 = call "Calc phase increase and offset.vi"("# of DDS"=2, "fclk (MHz)"=250.0 ("fclk (800MHz)"), "f_generated (MHz)"=w234) -> ("Phase out"=w235:fxp<+,64,64>[])  [unwired: 6 in, 2 out]
              }
              frame Enabled {
                n138 = call "Calc phase increase and offset.vi"("# of DDS"=4, "fclk (MHz)"=500.0 ("fclk (800MHz)"), "f_generated (MHz)"=w238) -> ("Phase out"=w239:fxp<+,64,64>[])  [unwired: 6 in, 2 out]
              }
              frame Disabled {
              }
            }
            n139 = Unbundle By Name(w231) -> ("FPGA ref"=w233:T14)
            n140 = xnode "Read/Write Control"("FPGA VI Reference In"=w233, "Phase output"=w227) -> ("FPGA VI Reference Out"=w232:T14, "error out"=w228:errorcluster)  [unwired: 1 in]
            n141 = flat-sequence {
              tunnel: w228 -> [_]
              frame #0 {
              }
            }
            n142 = Bundle By Name(cluster=w231, "FPGA ref"=w232) -> (w230:T17)
          }
          event "Output delay", "Output delay delta": Value Change {
            n143 = event-data() -> ()  [unwired: 1 in, 6 out]
            n144 = local read "Mixer freq [MHz]"() -> (w242:dbl)
            n145 = call "SetDelay.vi"("Mixer freq [MHz]"=w242, "Output delay delta"="Output delay delta", "Output delay"="Output delay", "scope in"=w246) -> ("scope out"=w245:T17)  [unwired: 7 in]
          }
          event "Fequency [kHz]", "a", "b": Value Change {
            n146 = event-data() -> ()  [unwired: 1 in, 6 out]
            n147 = disable-structure shown="Enabled" {
              disable-tunnel: w251 -> [w256 w257]
              disable-tunnel: [w255 w257] -> w250
              disable-tunnel: "Fequency [kHz]" -> [w254 _]
              disable-tunnel: "a" -> [w253 _]
              disable-tunnel: "b" -> [w252 _]
              frame Enabled {
                n148 = call "SetAmplitudeModulation.vi"("b_am"=w252, "a_am"=w253, "Am freq [kHz]"=w254, "scope in"=w256) -> ("scope out"=w255:T17)  [unwired: 7 in]
              }
              frame Disabled {
              }
            }
          }
          event "ch0 DC offset": Value Change {
            n149 = event-data() -> ()  [unwired: 1 in, 6 out]
            n150 = Unbundle By Name(w271) -> ("FPGA ref"=w263:T14)
            n151 = Divide(x=32768, y=5) -> (x/y=w267:dbl)
            n152 = Multiply(x="ch0 DC offset", y=w267) -> (x*y=w265:dbl)
            n153 = Round To Nearest(number=w265) -> (nearest integer value=w264:dbl)
            n154 = To Word Integer(number=w264) -> (16bit integer=w262:i16)
            n155 = xnode "Reinterpret Number"("x"=w262) -> ("y"=w261:fxp<+/-,16,14>)
            n156 = xnode "Reinterpret Number"("x"=w261) -> ("y"=w260:fxp<+,16,16>)
            n157 = call "Write 16bit value.vi"("value"=w260, "FPGA Setting"=fpga_settings."DC_offs 0", "FPGA ref"=w263) -> ("FPGA VI Reference Out"=w259:T14)  [unwired: 8 in]
            n158 = Bundle By Name(cluster=w271, "FPGA ref"=w259) -> (w270:T17)
          }
          event "ch1 DC offset": Value Change {
            n159 = event-data() -> ()  [unwired: 1 in, 6 out]
            n160 = Unbundle By Name(w285) -> ("FPGA ref"=w278:T14)
            n161 = Divide(x=32768, y=5) -> (x/y=w281:dbl)
            n162 = Multiply(x="ch1 DC offset", y=w281) -> (x*y=w280:dbl)
            n163 = Round To Nearest(number=w280) -> (nearest integer value=w279:dbl)
            n164 = To Word Integer(number=w279) -> (16bit integer=w277:i16)
            n165 = xnode "Reinterpret Number"("x"=w277) -> ("y"=w276:fxp<+/-,16,14>)
            n166 = xnode "Reinterpret Number"("x"=w276) -> ("y"=w275:fxp<+,16,16>)
            n167 = call "Write 16bit value.vi"("value"=w275, "FPGA Setting"=fpga_settings."DC_offs 1", "FPGA ref"=w278) -> ("FPGA VI Reference Out"=w274:T14)  [unwired: 8 in]
            n168 = Bundle By Name(cluster=w285, "FPGA ref"=w274) -> (w284:T17)
          }
          event Value Change {
            n169 = event-data() -> ()  [unwired: 1 in, 6 out]
            n170 = Unbundle By Name(w289) -> ("FPGA ref"=w291:T14)
            n171 = property on="Rumode" class="Bool (strict)"("Val(Sgnl)"=FALSE ("Value (Signaling)")) -> ()  [unwired: 2 in, 2 out]
            n172 = xnode "Read/Write Control"("FPGA VI Reference In"=w291, "Mode"="Mode") -> ("FPGA VI Reference Out"=w290:T14)  [unwired: 1 in, 1 out]
            n173 = Bundle By Name(cluster=w289, "FPGA ref"=w290, "data mode"="Mode") -> (w288:T17)
          }
          event Value Change {
            n174 = event-data() -> ()  [unwired: 1 in, 6 out]
            n175 = Bundle By Name(cluster=w293, "5782 Trigger"="Trigger") -> (w292:T17)
          }
          event "Samples per 5782 record": Value Change {
            n176 = event-data() -> ()  [unwired: 1 in, 6 out]
            n177 = Unbundle By Name(w296) -> ("FPGA ref"=w299:T14)
            n178 = xnode "Read/Write Control"("FPGA VI Reference In"=w299, "5782 record length"="Samples per 5782 record") -> ("FPGA VI Reference Out"=w298:T14)  [unwired: 1 in, 1 out]
            n179 = Bundle By Name(cluster=w296, "FPGA ref"=w298, "samples per record"="Samples per 5782 record") -> (w295:T17)
          }
          event "Singleshot": Value Change {
            n180 = event-data() -> ()  [unwired: 1 in, 6 out]
            n181 = local write "Rumode"(FALSE ("Rumode")) -> ()
            n182 = Bundle By Name(cluster=w308, "scope mode"=ScopeMode."Single") -> (w304:T17)
            n183 = call "ToggleContinousMode.vi"("Cont Acquisition"=FALSE, "scope in"=w304) -> ("scope out"=w303:T17)  [unwired: 8 in, 1 out]
            n184 = call "ToggleAqcuisitionRunning_5782.vi"("Acquisition running"=TRUE, "scope in"=w303) -> ("scope out"=w306:T17)  [unwired: 8 in, 1 out]
            n185 = call "SendSWtrigger_5782.vi"("scope in"=w306) -> ("scope out"=w301:T17)  [unwired: 9 in, 1 out]
            n186 = Bundle By Name(cluster=w301, "last phase"=dbl[] [0.0, 0.0]) -> (w300:T17)
          }
          event "Rumode": Value Change {
            n187 = event-data() -> ()  [unwired: 1 in, 6 out]
            n188 = case shown="\"Triggered\"" "Trigmode" {
              tunnel: [ScopeMode."Running" ("scope mode") ScopeMode."Continuous" ("scope mode")] -> w312
              frame "Triggered" {
              }
              frame "Continuous" {
              }
            }
            n189 = Select(t=w312, s="Rumode", f=ScopeMode."Stopped" ("scope mode")) -> (s? t:f=w316:T18)
            n190 = Bundle By Name(cluster=w317, "last phase"=dbl[] [0.0, 0.0], "scope mode"=w316) -> (w315:T17)
            n191 = case shown="\"Single\", \"Running\"" w316 {
              tunnel: w315 -> [w324 w331 w335]
              tunnel: [w325 w329 w336] -> w314
              frame "Single", "Running" {
                n192 = call "ToggleContinousMode.vi"("Cont Acquisition"=FALSE, "scope in"=w324) -> ("scope out"=w322:T17)  [unwired: 8 in, 1 out]
                n193 = call "ToggleAqcuisitionRunning_5782.vi"("Acquisition running"=TRUE, "scope in"=w322) -> ("scope out"=w326:T17)  [unwired: 8 in, 1 out]
                n194 = call "SendSWtrigger_5782.vi"("scope in"=w326) -> ("scope out"=w325:T17)  [unwired: 9 in, 1 out]
              }
              frame "Continuous" {
                n195 = call "ToggleAqcuisitionRunning_5782.vi"("Acquisition running"=TRUE, "scope in"=w331) -> ("scope out"=w330:T17)  [unwired: 8 in, 1 out]
                n196 = call "ToggleContinousMode.vi"("Cont Acquisition"=TRUE ("Acquisition running"), "scope in"=w330) -> ("scope out"=w329:T17)  [unwired: 8 in, 1 out]
              }
              frame "Stopped" {
                n197 = call "ToggleContinousMode.vi"("Cont Acquisition"=FALSE, "scope in"=w335) -> ("scope out"=w333:T17)  [unwired: 8 in, 1 out]
                n198 = call "ToggleAqcuisitionRunning_5782.vi"("Acquisition running"=FALSE, "scope in"=w333) -> ("scope out"=w336:T17)  [unwired: 8 in, 1 out]
              }
            }
          }
          event Value Change {
            n199 = event-data() -> ("CtlRef"=w340:refnum<vi>, "NewVal"=w338:bool)  [unwired: 1 in, 4 out]
            n200 = Search 1D Array(1D array=w341, element=w340) -> (index of element=w339:i32)  [unwired: 1 in]
            n201 = property on="Upper chart" class="WFChart (strict)"("Active Plot"=w339, "Plot.Visible?"=w338) -> ()  [unwired: 2 in, 2 out]
          }
          event Value Change {
            n202 = event-data() -> ("CtlRef"=w346:refnum<vi>, "NewVal"=w343:bool)  [unwired: 1 in, 4 out]
            n203 = Search 1D Array(1D array=w345, element=w346) -> (index of element=w344:i32)  [unwired: 1 in]
            n204 = property on="freqdata" class="WFGraph (strict)"("Active Plot"=w344, "Plot.Visible?"=w343) -> ()  [unwired: 2 in, 2 out]
            n205 = property on="Lower chart" class="WFChart (strict)"("Active Plot"=w344, "Plot.Visible?"=w343) -> ()  [unwired: 2 in, 2 out]
          }
          event User Event {
            n206 = event-data() -> ("Sender"=w352:string, "Variant"=w351:variant, "driver status"=w350:T13)  [unwired: 1 in, 5 out]
            n207 = Unbundle By Name(w349) -> ("RemoteConnection"=w354:refnum<class "RemoteConnection.lvclass">)
            n208 = call "HandleRemoteMessage.vi"("driver status"=w350, "Message data"=w351, "Sender"=w352, "RemoteConnection in"=w354) -> ("RemoteConnection out"=w353:refnum<class "RemoteConnection.lvclass">)  [unwired: 6 in, 1 out]
            n209 = Bundle By Name(cluster=w349, "RemoteConnection"=w353) -> (w348:T17)
          }
          event "stop": Value Change {
            n210 = event-data() -> ()  [unwired: 1 in, 6 out]
          }
          event Value Change {
            n211 = event-data() -> ()  [unwired: 1 in, 6 out]
            n212 = case shown="\"V\"" "Unit" {
              tunnel: ["V" "dBV" "V^2"] -> w359
              frame "V" {
              }
              frame "dBV" {
              }
              frame "V^2" {
              }
            }
            n213 = Concatenate Strings("Amplitude [", w359, "]") -> (w357:string)
            n214 = property on="freqdata" class="WFGraph (strict)"("YScale.NameLbl.Text"=w357) -> ()  [unwired: 2 in, 2 out]
          }
          event "#bins": Value Change {
            n215 = event-data() -> ()  [unwired: 1 in, 6 out]
            n216 = local read "Upper chart"() -> (w368:dbl[][])
            n217 = local read "Window"() -> (w369:T8)
            n218 = local read "Unit"() -> (w370:T7)
            n219 = call "calc FFT.vi"("#bins"="#bins", "dt"=1e-06, "Unit"=w370, "Window"=w369, "data"=w368) -> ("Power Spectrum / PSD"=w367:cluster{"f0":dbl, "df":dbl, "magnitude":dbl[]}[])  [unwired: 6 in]
            n220 = local write "freqdata"(w367) -> ()
          }
          event "Zoom time X", "Zoom time Y": Value Change {
            n221 = event-data() -> ()  [unwired: 1 in, 6 out]
            n222 = control-ref of="Upper chart"() -> (w375:refnum<vi>)
            n223 = call "setZoomTool.vi"("Zoom Y"="Zoom time Y", "Zoom  X"="Zoom time X", "reference"=w375) -> ()  [unwired: 9 in]
            n224 = call "setZoomTool.vi"("Zoom Y"="Zoom time Y", "Zoom  X"="Zoom time X") -> ()  [unwired: 10 in]
          }
          event "Zoom freq Y", "Zoom freq X": Value Change {
            n225 = event-data() -> ()  [unwired: 1 in, 6 out]
            n226 = control-ref of="Lower chart"() -> (w380:refnum<vi>)
            n227 = control-ref of="Lower graph"() -> (w379:refnum<vi>)
            n228 = control-ref of="freqdata"() -> (w381:refnum<vi>)
            n229 = call "setZoomTool.vi"("Zoom Y"="Zoom freq Y", "Zoom  X"="Zoom freq X", "reference"=w381) -> ()  [unwired: 9 in]
            n230 = call "setZoomTool.vi"("Zoom Y"="Zoom freq Y", "Zoom  X"="Zoom freq X", "reference"=w380) -> ()  [unwired: 9 in]
            n231 = call "setZoomTool.vi"("Zoom Y"="Zoom freq Y", "Zoom  X"="Zoom freq X", "reference"=w379) -> ()  [unwired: 9 in]
          }
          event Value Change {
            w391 = dbl[][] [] ("History Data")
            n232 = event-data() -> ()  [unwired: 1 in, 6 out]
            n233 = case shown="\"Time and Frequency\", Default" "Display" {
              tunnel: ["deltaF" _] -> w386
              frame "Time and Frequency", Default {
              }
              frame "Phase and Magnitude" {
              }
            }
            n234 = property on="Upper chart" class="WFChart (strict)"("History Data"=w391) -> ()  [unwired: 2 in, 2 out]
            n235 = property on="Lower chart" class="WFChart (strict)"("History Data"=w391) -> ()  [unwired: 2 in, 2 out]
            n236 = local write "freqdata"(cluster{"f0":dbl, "df":dbl, "magnitude":dbl[]}[] [] ("freqdata")) -> ()
            n237 = call "UpdateGraphs.vi"("Buffer mode"="Buffer", "Display mode"="Display", "Graph_refs"=w392) -> ()  [unwired: 9 in]
            n238 = property on="Zoom time X" class="Bool (strict)"("Val(Sgnl)"=TRUE ("Value (Signaling)")) -> ()  [unwired: 2 in, 2 out]
            n239 = property on="Upper chart" class="WFChart (strict)"("Active Plot"=u32 3, "Plot.Visible?"=w386) -> ()  [unwired: 2 in, 2 out]
            n240 = Bundle By Name(cluster=w385, "last phase"=dbl[] [0.0, 0.0]) -> (w383:T17)
          }
        }
      }
      "stop 2" <- w108
    }
    frame Error {
    }
  }
  n241 = Unregister For Events(event registration refnum=w68) -> ()  [unwired: 1 in, 1 out]
  n242 = Unbundle By Name(w4) -> ("FPGA ref"=w6:T14, "RemoteConnection"=w5:refnum<class "RemoteConnection.lvclass">)
  n243 = flat-sequence {
    tunnel: w6 -> [w399]
    tunnel: w5 -> [w398]
    frame #0 {
      n244 = call "Close.vi"("RemoteConnection in"=w398) -> ()  [unwired: 9 in, 2 out]
      n245 = xnode "Close FPGA VI Reference"("FPGA VI Reference In"=w399) -> ()  [unwired: 1 in, 1 out]
      n246 = global write "global_stop.vi" "Stop"(TRUE ("Stop")) -> ()
    }
  }
